vi "configure.vi"(8 "error in (no error)":errorcluster, 11 "DL090201FrameScanTrajectory in":refnum<class "TrajectoryDL090201FrameScan.lvclass">) -> (0 "error out":errorcluster, 3 "DL090201FrameScanTrajectory out":refnum<class "TrajectoryDL090201FrameScan.lvclass">)   [LabVIEW 2010, in "TrajectoryDL090201FrameScan.lvclass"]
uses:
  TrajectoryDL090201FrameScan.lvclass
  TrajectoryDL090201FrameScan.lvclass/TrajectoryDL090201FrameScan.ctl
  common/classes/ErrorController/ErrorController/class_data.vi
  common/classes/GenericComponent/GenericComponent/GenericComponent.lvclass
  common/classes/ErrorController/ErrorController/ErrorController.lvclass
panel:
  in  "y retrace lines":i32 min=0
  out "Configuration":string
  in  "x retrace fraction":dbl
  in  "x scan cut-off fraction":dbl
  in  "save":bool
  in  "cancel":bool
  # "Configure DL090201FrameScanTrajectory"
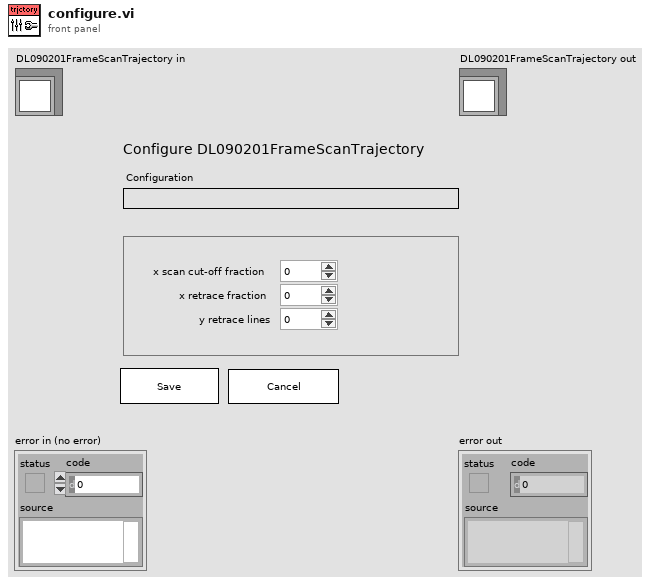
[diagram p1: front panel]
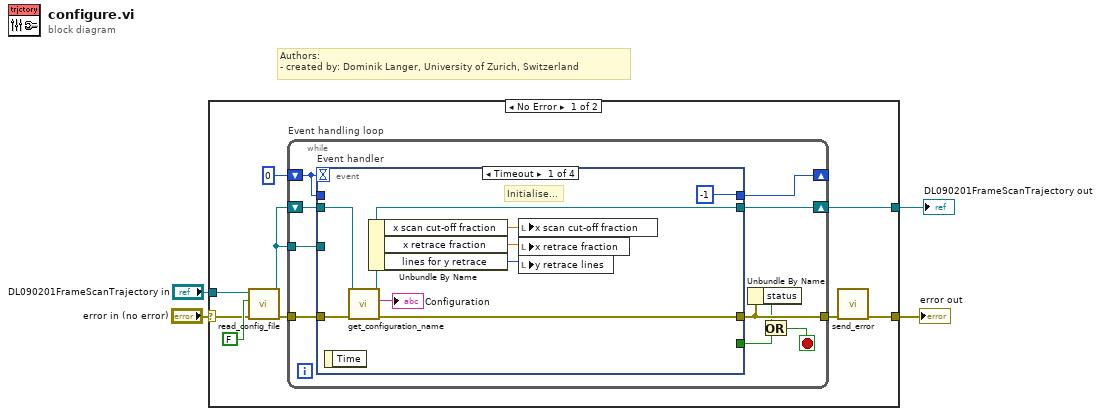
[diagram p0: block diagram]
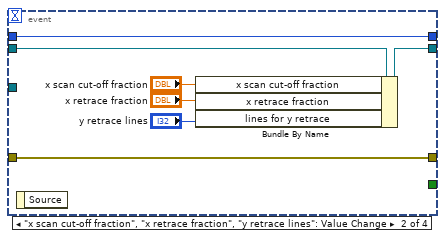
[diagram p2: hidden frame]
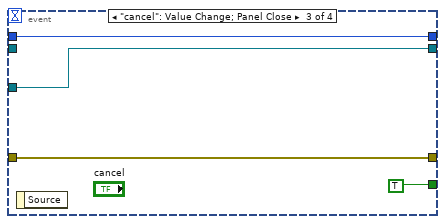
[diagram p3: hidden frame]
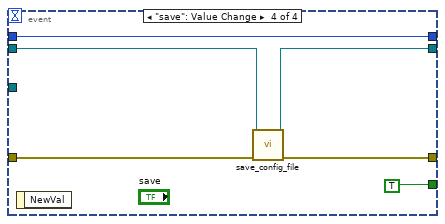
[diagram p4: hidden frame]
diagram:
  # "Authors: \n- created by: Dominik Langer, University of Zurich, Switzerland"
  n1 = case shown="No Error" "error in (no error)" {
    selector: "error in (no error)" -> [w10 w51]
    tunnel: [w7 w51] -> w3
    tunnel: [w13 w50] -> w1
    tunnel: "DL090201FrameScanTrajectory in" -> [w8 w50]
    frame No Error {
      n2 = call-dynamic "read_config_file.vi"("error in (no error)"=w10, "force load?"=FALSE, "GenericPlugin in"=w8) -> ("error out"=w9:errorcluster, "GenericPlugin out"=w5:refnum<class "TrajectoryDL090201FrameScan.lvclass">)  [unwired: 7 out]
      n3 = while "Event handling loop" {
        shift-right: [w21] -> w13
        shift-left: w5 -> [w22]
        shift-right: [w19] -> _
        shift-left: 0 -> [w20]
        tunnel: w9 -> [w23]
        tunnel: [w18] -> w6
        tunnel: w5 -> [w14]
        stop <- w15 stop-if-true
        n4 = event "Event handler" shown="[0] Timeout" {
          selector: _ -> [_ _ _ _]
          dyn-events: _ -> [_ _ _ _]
          timeout: w20 -> [_ _ _ _]
          tunnel: w23 -> [w29 w39 w43 w49]
          tunnel: [w28 w39 w43 w48] -> w18
          tunnel: w22 -> [w27 w37 _ w44]
          tunnel: [w26 w36 w40 w47] -> w21
          tunnel: [_ _ TRUE TRUE] -> w17
          tunnel: [-1 w38 w41 w45] -> w19
          tunnel: w20 -> [_ w38 w41 w45]
          tunnel: w14 -> [_ _ w40 _]
          event Timeout {
            # "Initialise..."
            n5 = event-data() -> ()  [unwired: 2 out]
            n6 = call "get_configuration_name.vi"("error in (no error)"=w29, "GenericPlugin.lvclass in"=w27) -> ("error out"=w28:errorcluster, "configuration name"=→"Configuration":string, "GenericPlugin.lvclass out"=w26:refnum<class "TrajectoryDL090201FrameScan.lvclass">)  [unwired: 7 in]
            n7 = Unbundle By Name(w26) -> ("x scan cut-off fraction"=w31:dbl, "x retrace fraction"=w30:dbl, "lines for y retrace"=w24:i32)
            n8 = local write "x scan cut-off fraction"(w31) -> ()
            n9 = local write "x retrace fraction"(w30) -> ()
            n10 = local write "y retrace lines"(w24) -> ()
          }
          event "x scan cut-off fraction", "x retrace fraction", "y retrace lines": Value Change {
            n11 = event-data() -> ()  [unwired: 2 out]
            n12 = Bundle By Name(cluster=w37, "x scan cut-off fraction"="x scan cut-off fraction", "x retrace fraction"="x retrace fraction", "lines for y retrace"="y retrace lines") -> (w36:refnum<class "TrajectoryDL090201FrameScan.lvclass">)
          }
          event "cancel": Value Change; Panel Close {
            n13 = event-data() -> ()  [unwired: 2 out]
          }
          event "save": Value Change {
            n14 = event-data() -> ()  [unwired: 2 out]
            n15 = call-dynamic "save_config_file.vi"("error in (no error)"=w49, "GenericPlugin in"=w44) -> ("error out"=w48:errorcluster, "GenericPlugin out"=w47:refnum<class "TrajectoryDL090201FrameScan.lvclass">)  [unwired: 2 in, 6 out]
          }
        }
        n16 = Unbundle By Name(w18) -> ("status"=w16:bool)
        n17 = Or(x=w16, y=w17) -> (x .or. y?=w15:bool)
      }
      n18 = call "send_error.vi"("error in (no error)"=w6) -> ("error out"=w7:errorcluster)  [unwired: 10 in]
    }
    frame Error {
    }
  }
  "error out" <- w3
  "DL090201FrameScanTrajectory out" <- w1
